vi "Write Buffer Type.vi"(8 "error in (no error)":errorcluster, 10 "Buffer Type":T1, 11 "CIF_CIPC_Chn in":refnum<class "CIF_CIPC_Chn.lvclass">) -> (0 "error out":errorcluster, 3 "CIF_CIPC_Chn out":refnum<class "CIF_CIPC_Chn.lvclass">)   [LabVIEW 2021, in "CIF_CIPC_Chn.lvclass"]
uses:
  CIF_CIPC_Chn.lvclass
  CIF_CIPC_Chn.lvclass/CIF_CIPC_Chn.ctl
  Typedef/Buffer Type.ctl
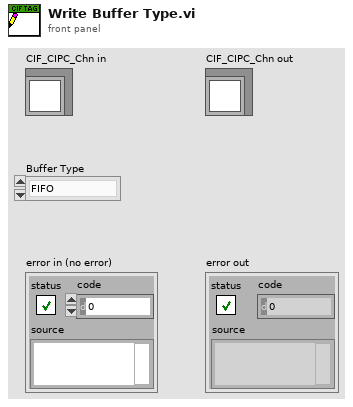
[diagram p1: front panel]
types:
  T1 = typedef "CIF_CIPC_Chn.lvclass/Buffer Type.ctl" = enum16{"FIFO", "Backpressure FIFO"}
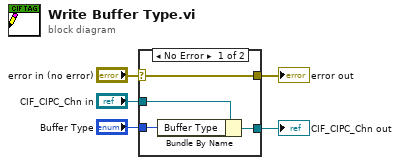
[diagram p0: block diagram]
diagram:
  n1 = case shown="No Error" "error in (no error)" {
    selector: "error in (no error)" -> [w9 w10]
    tunnel: [w9 w10] -> w4
    tunnel: [w7 w11] -> w2
    tunnel: "CIF_CIPC_Chn in" -> [w8 w11]
    tunnel: "Buffer Type" -> [w6 _]
    frame No Error {
      n2 = Bundle By Name(cluster=w8, "Buffer Type"=w6) -> (w7:refnum<class "CIF_CIPC_Chn.lvclass">)
    }
    frame Error {
    }
  }
  "error out" <- w4
  "CIF_CIPC_Chn out" <- w2
